vi "graph.vi"() -> ()   [LabVIEW 2020]
panel:
  in  "Amplitude":dbl=1.0
  in  "Frequency":dbl=10.1
  in  "stop":bool
  out "Waveform Chart":dynamicdata(graph)
  in  "Cluster":T1
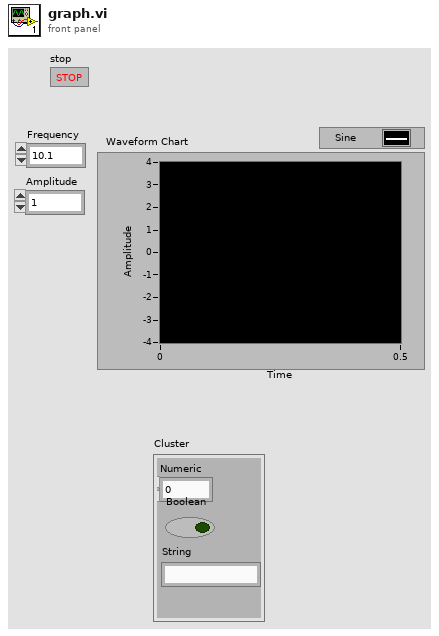
[diagram p1: front panel]
types:
  T1 = cluster{"Numeric":dbl, "Boolean":bool, "String":string}
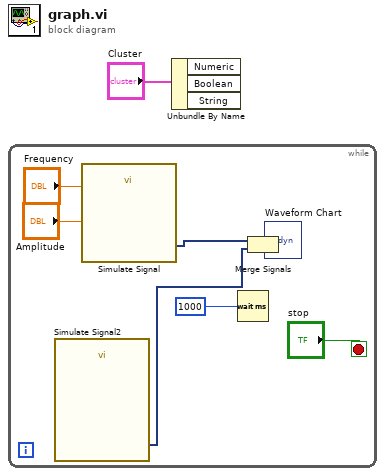
[diagram p0: block diagram]
diagram:
  n1 = while {
    stop <- "stop" stop-if-true
    n2 = call "Simulate Signal2"() -> ("Square"=w2:dynamicdata)  [unwired: 14 in, 1 out]
    n3 = call "Simulate Signal"("Frequency"="Frequency", "Amplitude"="Amplitude") -> ("Sine"=w8:dynamicdata)  [unwired: 12 in, 1 out]
    n4 = Wait (ms)(milliseconds to wait=u32 1000 ("millisecond timer value")) -> ()  [unwired: 1 out]
    n5 = Merge Signals(w8, w2) -> (→"Waveform Chart":dynamicdata)
  }
  n6 = Unbundle By Name("Cluster") -> ()  [unwired: 3 out]
